vi "Periodic Tasks.vi"(8 "error in":errorcluster) -> ()   [LabVIEW 2015]
doc: "This VI runs in parallel to other tasks. It can contain as many user-defined periodic loops as you need. These can carry out PID or other sorts of timed response."
uses:
  Robot Global Data.vi
  <vilib>/Rock Robotics/WPI/Utilities/WPI_GetSetVariantRefNum.vi
  <vilib>/Rock Robotics/WPI/RobotDrive/WPI_RobotDriveArcadeDrive_Standard(NoSaturation).vi
  <vilib>/Rock Robotics/Network Tables/NT Write Number.vi
  navX Library v2/navX Library v2.lvlib
panel:
  out "gyro":dbl
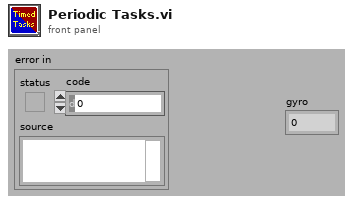
[diagram p1: front panel]
types:
  T1 = typedef "WPI_AnalogChannelDevRef.ctl" = cluster{"DevStatus":errorcluster, "Analog Channel":T2}
  T2 = typedef "FPGA_AIChannel.ctl" = enum8{"AI 0", "AI 1", "AI 2", "AI 3", "AI MXP 0", "AI MXP 1", "AI MXP 2", "AI MXP 3", "Invalid"}
  T3 = typedef "navX Library v2.lvlib/Z900_navX_DeviceTypeDef.ctl" = cluster{"Interface":cluster{"Protocol":T4, "Update Rate (4Hz-60Hz)":u8, "navX Open TypeDef":variant}, "Notify Packet":refnum<notifier>, "Loop VI Refnum":refnum<vi>, "Ready to Close Occurrence Refnum":refnum<k4>}
  T4 = typedef "navX Library v2.lvlib/Z900_navX_ProtocolTypeDef.ctl" = enum16{"SERIAL", "I2C", "SPI"}
  T5 = cluster{"Yaw":dbl, "Roll":dbl, "Pitch":dbl, "Heading":dbl, "Fused Heading":dbl}
  T6 = typedef "WPI_MotorControlDeviceRef.ctl" = cluster{"DeviceStatus":errorcluster, "Type":T7, "PWM":cluster{"PWM Channel":T8, "DeadBand":T9}, "CAN":cluster{"Device Number":u8, "Control Mode":T10, "Semaphore":T11, "Max Vout":dbl, "TalonSRX Control Mode":T12}, "Invert":bool}
  T7 = typedef "WPI_MotorControlType.ctl" = enum16{"PWM", "CAN", "CANTalonSRX"}
  T8 = typedef "FPGA_DIOPWMChannel.ctl" = enum8{"PWM 0", "PWM 1", "PWM 2", "PWM 3", "PWM 4", "PWM 5", "PWM 6", "PWM 7", "PWM 8", "PWM 9", "PWM MXP 0", "PWM MXP 1", "PWM MXP 2", "PWM MXP 3", "PWM MXP 4", "PWM MXP 5", "PWM MXP 6", "PWM MXP 7", "PWM MXP 8", "PWM MXP 9", "Invalid"}
  T9 = typedef "WPI_PWMDeadband.ctl" = cluster{"Name":string, "maxPositivePwm":i32, "minPositivePwm":i32, "centerPwm":i32, "maxNegativePwm":i32, "minNegativePwm":i32, "angularRange":u16}
  T10 = typedef "WPI_CANJaguar_ControlMode.ctl" = enum8{"Percent VBus", "Current", "Speed", "Position", "Voltage"}
  T11 = typedef "Semaphore RefNum" = refnum<k1>
  T12 = typedef "WPI_CANTalonSRX_APIControlMode.ctl" = enum8{"Percent VBus", "Speed", "Position", "Slave", "Unchanged / Invalid", "Voltage Compensation", "Current", "Motion Profile"}
  T13 = typedef "WPI_ServoDeviceRef.ctl" = cluster{"DeviceStatus":errorcluster, "PWM Channel":T8, "DeadBand":T9}
  T14 = typedef "WPI_RobotDriveDevRef.ctl" = cluster{"DevStatus":errorcluster, "Motors[]":T6[], "Square Inputs":bool, "Max Output":dbl}
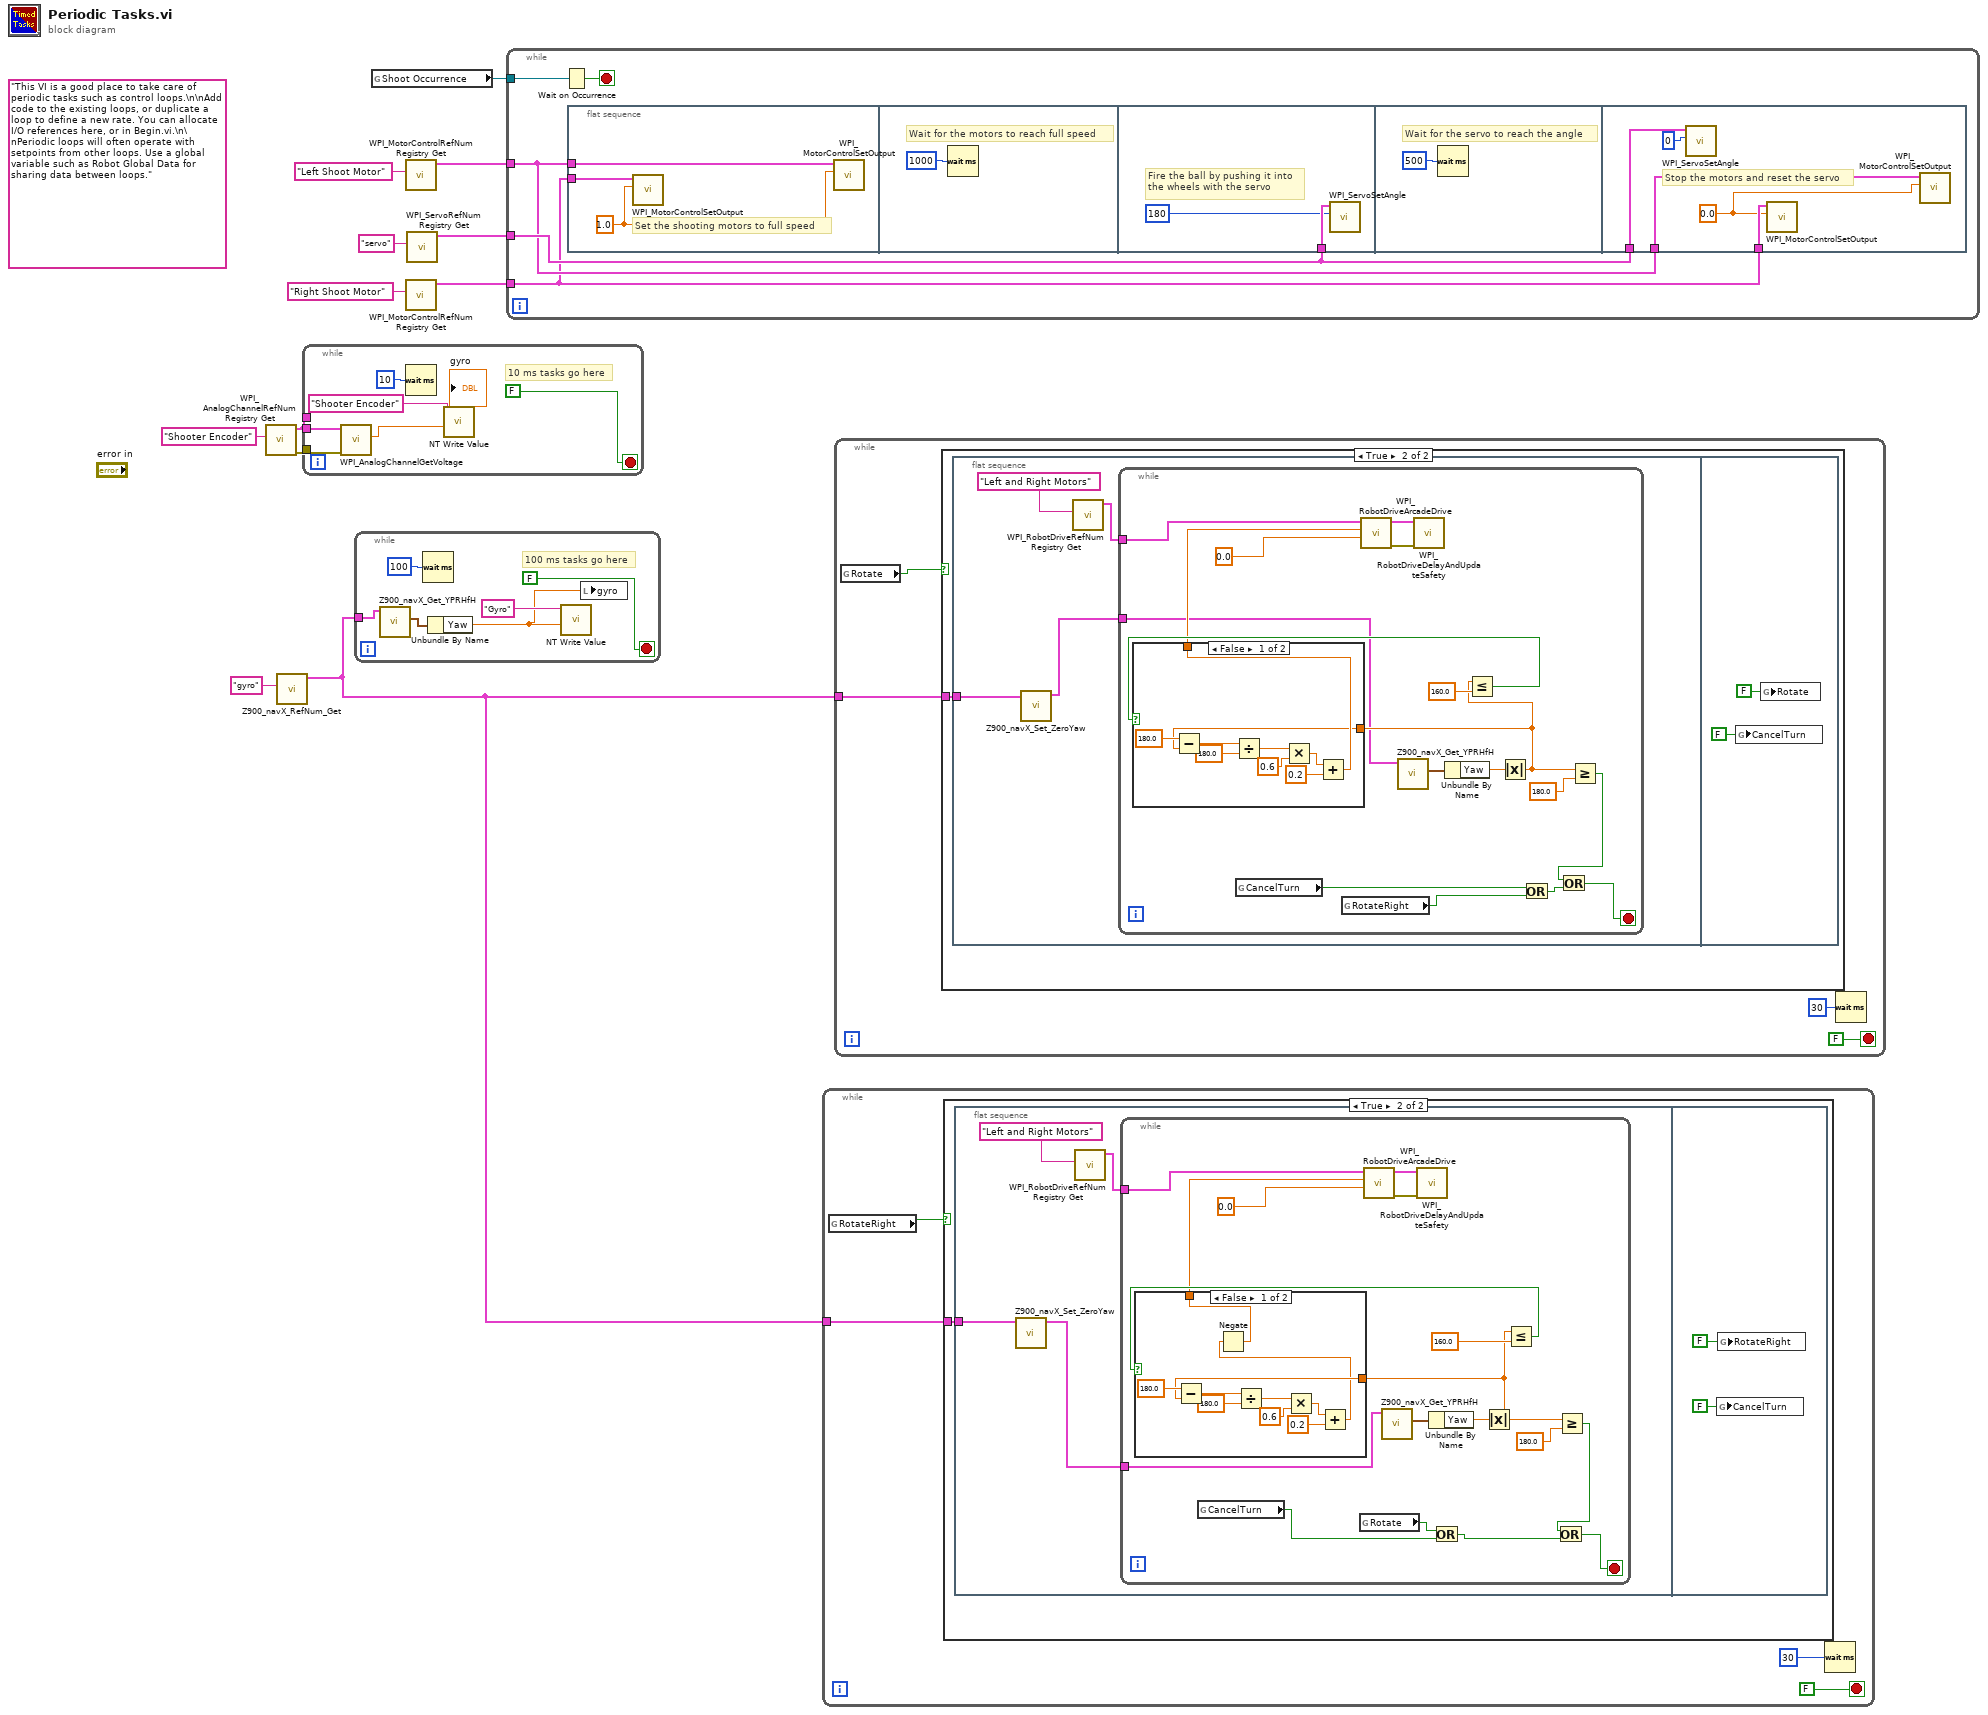
[diagram p0: block diagram]
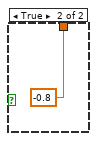
[diagram p3: hidden frame]
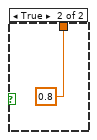
[diagram p5: hidden frame]
diagram:
  (unwired) "This VI is a good place to take care of periodic tasks such as control loops.\n\nAdd code to the existing loops, or duplicate a loop to define a new rate. You can allocate I/O references here, or in Begin.vi.\n\nPeriodic loops will often operate with setpoints from other loops. Use a global variable such as Robot Global Data for sharing data between loops."
  n1 = call <vilib>:"WPI_AnalogChannelRefNum Registry Get.vi"("refnum name"="Shooter Encoder") -> ("error out"=w4:errorcluster, "AIDeviceRef"=w5:T1)  [unwired: 9 in]
  n2 = call "Z900_navX_RefNum_Get.vi"("refnum name"="gyro") -> ("navX Device"=w7:T3)  [unwired: 9 in, 1 out]
  n3 = while {
    tunnel: w5 -> [_]
    tunnel: w5 -> [w15]
    tunnel: w4 -> [w13]
    stop <- FALSE stop-if-true
    # "10 ms tasks go here"
    n4 = call <vilib>:"WPI_AnalogChannelGetVoltage.vi"("error in (no error)"=w13, "AIDeviceRef"=w15) -> ("Voltage"=w14:dbl)  [unwired: 7 in, 2 out]
    n5 = Wait (ms)(milliseconds to wait=u32 10) -> ()  [unwired: 1 out]
    n6 = call-poly <vilib>:"NT Write Value.vi"("Numeric"=w14, "Name"="Shooter Encoder") -> ()  [unwired: 9 in, 1 out]
  }
  n7 = while {
    tunnel: w7 -> [w20]
    stop <- FALSE stop-if-true
    # "100 ms tasks go here"
    n8 = call "Z900_navX_Get_YPRHfH.vi"("navX Device"=w20) -> ("YRPHfH"=w21:T5)  [unwired: 7 in, 3 out]
    n9 = Wait (ms)(milliseconds to wait=u32 100) -> ()  [unwired: 1 out]
    n10 = Unbundle By Name(w21) -> ("Yaw"=w19:dbl)
    n11 = call-poly <vilib>:"NT Write Value.vi"("Numeric"=w19, "Name"="Gyro") -> ()  [unwired: 9 in, 1 out]
    n12 = local write "gyro"(w19) -> ()
  }
  n13 = global read "Robot Global Data.vi" "Shoot Occurrence"() -> (w10:refnum<k4>)
  n14 = call <vilib>:"WPI_MotorControlRefNum Registry Get.vi"("refnum name"="Left Shoot Motor") -> ("MotorControlDevRef"=w1:T6)  [unwired: 9 in, 1 out]
  n15 = call <vilib>:"WPI_MotorControlRefNum Registry Get.vi"("refnum name"="Right Shoot Motor") -> ("MotorControlDevRef"=w3:T6)  [unwired: 9 in, 1 out]
  n16 = call <vilib>:"WPI_ServoRefNum Registry Get.vi"("refnum name"="servo") -> ("ServoDeviceRef"=w2:T13)  [unwired: 9 in, 1 out]
  n17 = while {
    tunnel: w3 -> [w25]
    tunnel: w1 -> [w26]
    tunnel: w10 -> [w28]
    tunnel: w2 -> [w27]
    stop <- w29 stop-if-true
    n18 = Wait on Occurrence(2:w28) -> (0:w29:bool)  [unwired: 2 in]
    n19 = flat-sequence {
      tunnel: w25 -> [w31]
      tunnel: w26 -> [w30]
      tunnel: w27 -> [w35]
      tunnel: w27 -> [w40]
      tunnel: w26 -> [w39]
      tunnel: w25 -> [w38]
      frame #0 {
        w32 = 1.0 ("Output")
        # "Set the shooting motors to full speed"
        n20 = call <vilib>:"WPI_MotorControlSetOutput.vi"("Output"=w32, "MotorControlDevRef"=w31) -> ()  [unwired: 7 in, 3 out]
        n21 = call <vilib>:"WPI_MotorControlSetOutput.vi"("Output"=w32, "MotorControlDevRef"=w30) -> ()  [unwired: 7 in, 3 out]
      }
      frame #1 {
        # "Wait for the motors to reach full speed"
        n22 = Wait (ms)(milliseconds to wait=u32 1000) -> ()  [unwired: 1 out]
      }
      frame #2 {
        # "Fire the ball by pushing it into the wheels with the servo"
        n23 = call <vilib>:"WPI_ServoSetAngle.vi"("Angle"=180, "ServoDeviceRef"=w35) -> ()  [unwired: 8 in, 2 out]
      }
      frame #3 {
        # "Wait for the servo to reach the angle"
        n24 = Wait (ms)(milliseconds to wait=u32 500) -> ()  [unwired: 1 out]
      }
      frame #4 {
        w37 = 0.0 ("Output")
        # "Stop the motors and reset the servo"
        n25 = call <vilib>:"WPI_ServoSetAngle.vi"("Angle"=0, "ServoDeviceRef"=w40) -> ()  [unwired: 8 in, 2 out]
        n26 = call <vilib>:"WPI_MotorControlSetOutput.vi"("Output"=w37, "MotorControlDevRef"=w38) -> ()  [unwired: 7 in, 3 out]
        n27 = call <vilib>:"WPI_MotorControlSetOutput.vi"("Output"=w37, "MotorControlDevRef"=w39) -> ()  [unwired: 7 in, 3 out]
      }
    }
  }
  n28 = while {
    tunnel: w7 -> [w42]
    stop <- FALSE stop-if-true
    n29 = global read "Robot Global Data.vi" "RotateRight"() -> (w45:bool)
    n30 = case shown="True" w45 {
      tunnel: w42 -> [_ w46]
      frame False {
      }
      frame True {
        n31 = flat-sequence {
          tunnel: w46 -> [w48]
          frame #0 {
            n32 = call "Z900_navX_Set_ZeroYaw.vi"("navX Device"=w48) -> ("navX Device"=w47:T3)  [unwired: 9 in, 1 out]
            n33 = call <vilib>:"WPI_RobotDriveRefNum Registry Get.vi"("refnum name"="Left and Right Motors") -> ("RobotDriveDevRef"=w49:T14)  [unwired: 1 in, 9 out]
            n34 = while {
              tunnel: w49 -> [w66]
              tunnel: w47 -> [w51]
              stop <- w56 stop-if-true
              n35 = global read "Robot Global Data.vi" "CancelTurn"() -> (w58:bool)
              n36 = global read "Robot Global Data.vi" "Rotate"() -> (w54:bool)
              n37 = call "Z900_navX_Get_YPRHfH.vi"("navX Device"=w51) -> ("YRPHfH"=w52:T5)  [unwired: 7 in, 3 out]
              n38 = Unbundle By Name(w52) -> ("Yaw"=w53:dbl)
              n39 = Or(x=w54, y=w58) -> (x .or. y?=w55:bool)
              n40 = Absolute Value(x=w53) -> (abs(x)=w59:dbl)
              n41 = Less Or Equal?(x=w59, y=160.0) -> (x <= y?=w61:bool)
              n42 = case shown="False" w61 {
                tunnel: [w69 -0.8 ("Y axis value")] -> w60
                tunnel: w59 -> [w70 _]
                frame False {
                  n43 = Subtract(x=180.0, y=w70) -> (x-y=w72:dbl)
                  n44 = Divide(x=w72, y=180.0) -> (x/y=w74:dbl)
                  n45 = Multiply(x=w74, y=0.6) -> (x*y=w76:dbl)
                  n46 = Add(x=w76, y=0.2) -> (x+y=w68:dbl)
                  n47 = Negate(x=w68) -> (-x=w69:dbl)
                }
                frame True {
                }
              }
              n48 = call-poly <vilib>:"WPI_RobotDriveArcadeDrive.vi"("Y axis value"=0.0, "X axis value"=w60, "RobotDriveDevRef"=w66) -> ("error out"=w64:errorcluster, "RobotDriveDevRef"=w63:T14)  [unwired: 6 in, 1 out]
              n49 = call <vilib>:"WPI_RobotDriveDelayAndUpdateSafety.vi"("error in (no error)"=w64, "RobotDriveDevRef"=w63) -> ()  [unwired: 8 in, 2 out]
              n50 = Greater Or Equal?(x=w59, y=180.0) -> (x >= y?=w57:bool)
              n51 = Or(x=w57, y=w55) -> (x .or. y?=w56:bool)
            }
          }
          frame #1 {
            n52 = global write "Robot Global Data.vi" "CancelTurn"(FALSE ("CancelTurn")) -> ()
            n53 = global write "Robot Global Data.vi" "RotateRight"(FALSE ("Rotate")) -> ()
          }
        }
      }
    }
    n54 = Wait (ms)(milliseconds to wait=u32 30) -> ()  [unwired: 1 out]
  }
  n55 = while {
    tunnel: w7 -> [w81]
    stop <- FALSE stop-if-true
    n56 = global read "Robot Global Data.vi" "Rotate"() -> (w84:bool)
    n57 = case shown="True" w84 {
      tunnel: w81 -> [_ w85]
      frame False {
      }
      frame True {
        n58 = flat-sequence {
          tunnel: w85 -> [w87]
          frame #0 {
            n59 = call "Z900_navX_Set_ZeroYaw.vi"("navX Device"=w87) -> ("navX Device"=w86:T3)  [unwired: 9 in, 1 out]
            n60 = call <vilib>:"WPI_RobotDriveRefNum Registry Get.vi"("refnum name"="Left and Right Motors") -> ("RobotDriveDevRef"=w88:T14)  [unwired: 1 in, 9 out]
            n61 = while {
              tunnel: w88 -> [w105]
              tunnel: w86 -> [w91]
              stop <- w95 stop-if-true
              n62 = global read "Robot Global Data.vi" "CancelTurn"() -> (w97:bool)
              n63 = global read "Robot Global Data.vi" "RotateRight"() -> (w93:bool)
              n64 = call "Z900_navX_Get_YPRHfH.vi"("navX Device"=w91) -> ("YRPHfH"=w90:T5)  [unwired: 7 in, 3 out]
              n65 = Unbundle By Name(w90) -> ("Yaw"=w92:dbl)
              n66 = Absolute Value(x=w92) -> (abs(x)=w98:dbl)
              n67 = Less Or Equal?(x=w98, y=160.0) -> (x <= y?=w100:bool)
              n68 = case shown="False" w100 {
                tunnel: [w108 0.8 ("Y axis value")] -> w99
                tunnel: w98 -> [w107 _]
                frame False {
                  n69 = Subtract(x=180.0, y=w107) -> (x-y=w110:dbl)
                  n70 = Divide(x=w110, y=180.0) -> (x/y=w112:dbl)
                  n71 = Multiply(x=w112, y=0.6) -> (x*y=w114:dbl)
                  n72 = Add(x=w114, y=0.2) -> (x+y=w108:dbl)
                }
                frame True {
                }
              }
              n73 = call-poly <vilib>:"WPI_RobotDriveArcadeDrive.vi"("Y axis value"=0.0, "X axis value"=w99, "RobotDriveDevRef"=w105) -> ("error out"=w103:errorcluster, "RobotDriveDevRef"=w102:T14)  [unwired: 6 in, 1 out]
              n74 = call <vilib>:"WPI_RobotDriveDelayAndUpdateSafety.vi"("error in (no error)"=w103, "RobotDriveDevRef"=w102) -> ()  [unwired: 8 in, 2 out]
              n75 = Or(x=w97, y=w93) -> (x .or. y?=w94:bool)
              n76 = Greater Or Equal?(x=w98, y=180.0) -> (x >= y?=w96:bool)
              n77 = Or(x=w96, y=w94) -> (x .or. y?=w95:bool)
            }
          }
          frame #1 {
            n78 = global write "Robot Global Data.vi" "CancelTurn"(FALSE ("CancelTurn")) -> ()
            n79 = global write "Robot Global Data.vi" "Rotate"(FALSE ("Rotate")) -> ()
          }
        }
      }
    }
    n80 = Wait (ms)(milliseconds to wait=u32 30) -> ()  [unwired: 1 out]
  }
